vi "DIO_PanelSim_Global.vi"(0 "menu":T4=enum."set value", 5 "DIO Channel":T3=enum."DIO 1", 7 "pulse Length":dbl format="%#.4f", 9 "Value Set":bool, 11 "error in (no error)":errorcluster, 12 "String Value":string) -> (10 "DIO new":T1={"type"="DIO", "device"="", "name"="", "data"={"<init"=FALSE, "<>value"=FALSE, "<pulse_length"=0, "<input"=FALSE}}, 15 "error out":errorcluster)   [LabVIEW 2019]
doc: "This is used to set and get the last motor output values. This is needed for simulation, since we cannot read these values from the hardware.\n\nThis software is licensed. Open the labview\\readme\\WPI Robotics Library Open Source License.txt file for more information."
uses:
  DIO data proto.ctl
  DIO proto.ctl
  <vilib>/Rock Robotics/SystemInterfaces/DIO/FPGA_DIOChannel.ctl
  DIO Update Ops.ctl
panel:
  out "All Values":T1[](array[typedef])
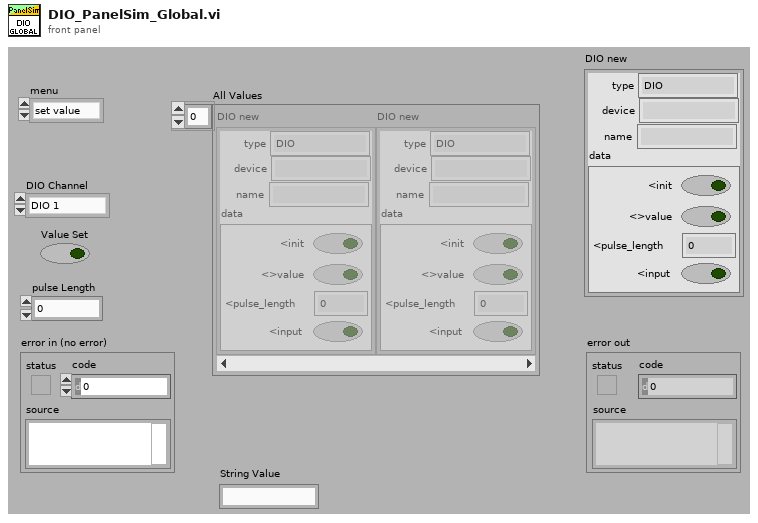
[diagram p1: front panel]
types:
  T1 = typedef "DIO proto.ctl" = cluster{"type":string, "device":string, "name":string, "data":T2}
  T2 = typedef "DIO data proto.ctl" = cluster{"<init":bool, "<>value":bool, "<pulse_length":i32, "<input":bool}
  T3 = typedef "FPGA_DIOChannel.ctl" = enum8{"DIO 0", "DIO 1", "DIO 2", "DIO 3", "DIO 4", "DIO 5", "DIO 6", "DIO 7", "DIO 8", "DIO 9", "DIO MXP 0", "DIO MXP 1", "DIO MXP 2", "DIO MXP 3", "DIO MXP 4", "DIO MXP 5", "DIO MXP 6", "DIO MXP 7", "DIO MXP 8", "DIO MXP 9", "DIO MXP 10", "DIO MXP 11", "DIO MXP 12", "DIO MXP 13", "DIO MXP 14", "DIO MXP 15", "SPI Port CS1", "SPI Port CS2", "SPI Port CS3", "SPI Port MISO", "SPI Port MOSI", "Invalid"}
  T4 = typedef "DIO Update Ops.ctl" = enum16{"set init", "set value", "set pulse_length", "set input", "get", "delete", "JSON update", "set name", "transmit initial", "reset"}
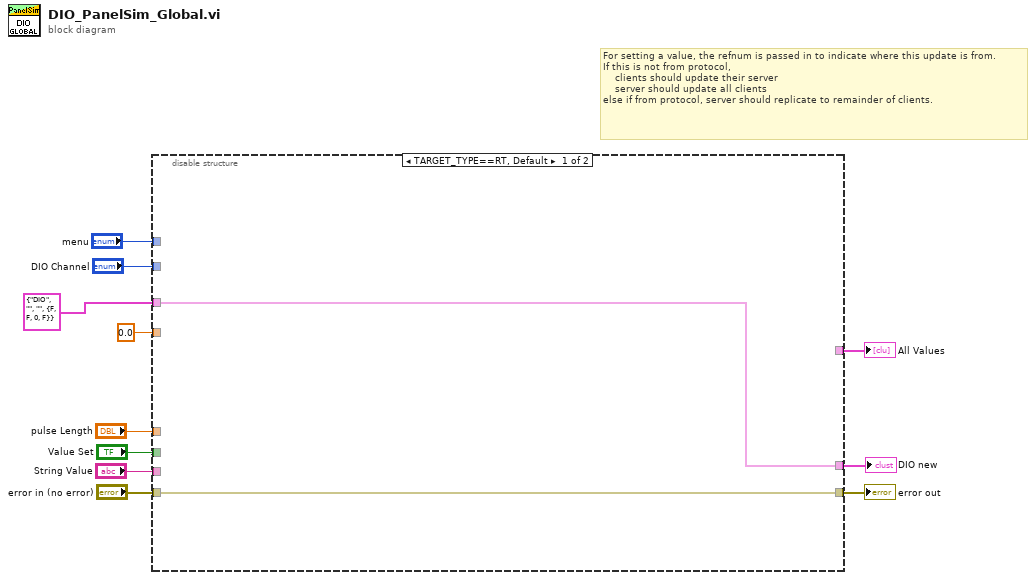
[diagram p0: block diagram]
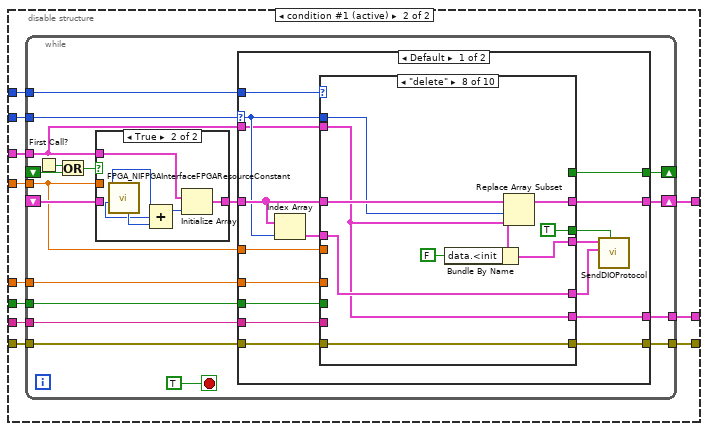
[diagram p2: hidden frame]
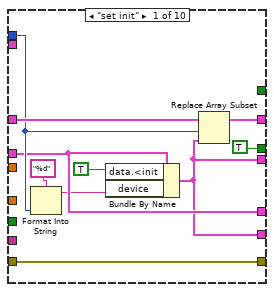
[diagram p3: hidden frame]
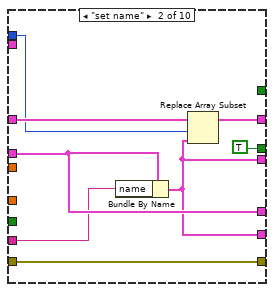
[diagram p4: hidden frame]
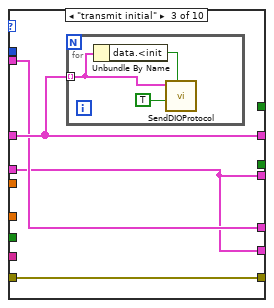
[diagram p5: hidden frame]
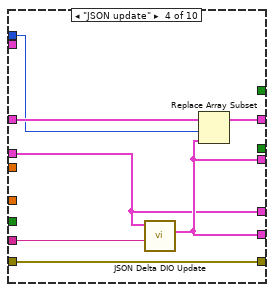
[diagram p6: hidden frame]
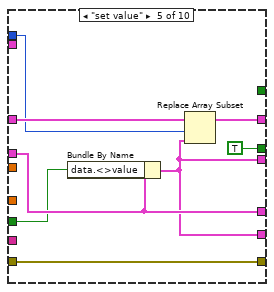
[diagram p7: hidden frame]
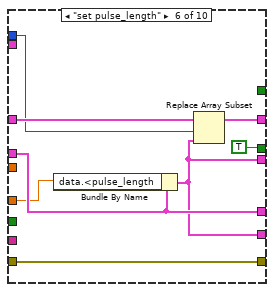
[diagram p8: hidden frame]
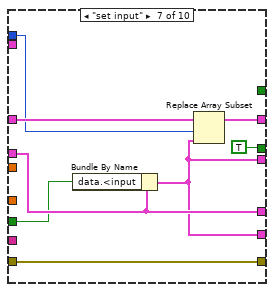
[diagram p9: hidden frame]
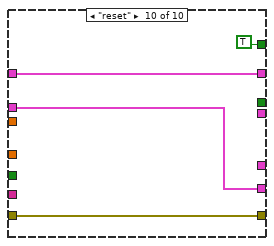
[diagram p11: hidden frame]
diagram:
  # "For setting a value, the refnum is passed in to indicate where this update is from.\nIf this is not from protocol,\n    clients should update their server\n    server should update all clients\nelse if from protocol, server should replicate to remainder of clients."
  n1 = disable-structure shown="TARGET_TYPE==RT, Default" {
    disable-tunnel: "menu" -> [_ w24]
    disable-tunnel: [w13 w23] -> w10
    disable-tunnel: "error in (no error)" -> [w13 w22]
    disable-tunnel: [_ w21] -> w8
    disable-tunnel: 0.0 ("Output") -> [_ w20]
    disable-tunnel: "Value Set" -> [_ w19]
    disable-tunnel: "DIO Channel" -> [_ w18]
    disable-tunnel: [w12 w17] -> w4
    disable-tunnel: T1 {"type"="DIO", "device"="", "name"="", "data"={"<init"=FALSE, "<>value"=FALSE, "<pulse_length"=0, "<input"=FALSE}} ("DIO new") -> [w12 w16]
    disable-tunnel: "String Value" -> [_ w15]
    disable-tunnel: "pulse Length" -> [_ w14]
    frame condition #0 {
    }
    frame condition #1 (active) {
      n2 = while {
        tunnel: w19 -> [w42]
        tunnel: w22 -> [w38]
        shift-right: [w41] -> w21
        shift-left: _ -> [w34]
        tunnel: [w40] -> w17
        tunnel: w24 -> [w39]
        tunnel: [w37] -> w23
        tunnel: w18 -> [w32]
        tunnel: w20 -> [w33]
        tunnel: w16 -> [w31]
        tunnel: w15 -> [w30]
        tunnel: w14 -> [w29]
        shift-right: [w25] -> _
        shift-left: _ -> [w26]
        stop <- TRUE stop-if-true
        n3 = First Call?() -> (First Call?: T/F=w27:bool)
        n4 = Or(x=w27, y=w26) -> (x .or. y?=w28:bool)
        n5 = case shown="True" w28 {
          tunnel: [w135 w141] -> w35
          tunnel: w34 -> [w135 _]
          tunnel: w33 -> [_ _]
          tunnel: w31 -> [_ w140]
          frame False {
          }
          frame True {
            n6 = call <vilib>:"FPGA_NIFPGAInterfaceFPGAResourceConstant.vi"() -> ("NumberOfDIOOnboard"=w138:u32, "NumberOfSPIDigitalPins"=w136:i32, "NumberOfSharedMXPpins"=w137:u32)  [unwired: 9 out]
            n7 = Compound Arithmetic op=ADD(w137, w136, w138) -> (w139:u32)
            n8 = Initialize Array(w140, w139) -> (w141:T1[])
          }
        }
        n9 = case shown="Default" w32 {
          selector: w32 -> [w51 _]
          tunnel: w42 -> [w59 _]
          tunnel: [w58 w134] -> w41
          tunnel: [w57 w132] -> w40
          tunnel: w39 -> [w56 _]
          tunnel: w38 -> [w55 w133]
          tunnel: [w54 w133] -> w37
          tunnel: w35 -> [w53 w134]
          tunnel: w33 -> [w52 _]
          tunnel: w31 -> [w49 w132]
          tunnel: w30 -> [w48 _]
          tunnel: w29 -> [w44 _]
          tunnel: [w43 _] -> w25
          frame Default {
            n10 = Index Array(array=w53, index=w51) -> (element=w50:T1)
            n11 = case shown="\"delete\"" w56 {
              tunnel: w59 -> [_ _ _ _ w93 _ w108 _ _ _]
              tunnel: [w69 w77 w80 w91 w99 w107 w115 w123 w127 w131] -> w58
              tunnel: w53 -> [w67 w75 w80 w89 w97 w105 w113 w124 w127 w131]
              tunnel: [w60 w71 w78 w87 w92 w101 w109 w117 w125 w129] -> w57
              tunnel: [w68 w76 w81 w90 w98 w106 w114 w122 w126 w130] -> w54
              tunnel: w55 -> [w68 w76 w81 w90 w98 w106 w114 w122 w126 w130]
              tunnel: w51 -> [w64 w73 _ w88 w95 w103 w111 w119 _ _]
              tunnel: w52 -> [_ _ _ _ _ _ _ _ _ _]
              tunnel: [w60 w71 w78 w87 w92 w101 w109 w118 _ _] -> w45
              tunnel: [w63 w72 w79 w85 w94 w102 w110 w120 _ _] -> w46
              tunnel: [TRUE TRUE _ _ TRUE TRUE TRUE TRUE _ _] -> w47
              tunnel: w50 -> [w63 w72 w78 w85 w94 w102 w110 w120 w125 w129]
              tunnel: w49 -> [_ _ w79 _ _ _ _ w117 _ _]
              tunnel: w48 -> [_ w70 _ w86 _ _ _ _ _ _]
              tunnel: w44 -> [_ _ _ _ _ w100 _ _ _ _]
              tunnel: [_ _ _ _ _ _ _ _ _ TRUE] -> w43
              frame "set init" {
                n12 = Format Into String(format string="%d", w64) -> (resulting string=w61:string)  [unwired: 2 in, 1 out]
                n13 = Bundle By Name(cluster=w63, "data.<init"=TRUE, "device"=w61) -> (w60:T1)
                n14 = Replace Array Subset(array=w67, new element=w60, index=w64) -> (w69:T1[])
              }
              frame "set name" {
                n15 = Bundle By Name(cluster=w72, "name"=w70) -> (w71:T1)
                n16 = Replace Array Subset(array=w75, new element=w71, index=w73) -> (w77:T1[])
              }
              frame "transmit initial" {
                n17 = for {
                  tunnel: w80 -> [w83] mode=indexing
                  n18 = Unbundle By Name(w83) -> ("data.<init"=w84:bool)
                  n19 = call "SendDIOProtocol.vi"("Send"=w84, "Initiualize"=TRUE, "DIO new"=w83) -> ()  [unwired: 9 in]
                }
              }
              frame "JSON update" {
                n20 = call "JSON Delta DIO Update.vi"("Delta JSON"=w86, "input"=w85) -> ("ouotput"=w87:T1)  [unwired: 8 in, 1 out]
                n21 = Replace Array Subset(array=w89, new element=w87, index=w88) -> (w91:T1[])
              }
              frame "set value" {
                n22 = Bundle By Name(cluster=w94, "data.<>value"=w93) -> (w92:T1)
                n23 = Replace Array Subset(array=w97, new element=w92, index=w95) -> (w99:T1[])
              }
              frame "set pulse_length" {
                n24 = Bundle By Name(cluster=w102, "data.<pulse_length"=w100) -> (w101:T1)
                n25 = Replace Array Subset(array=w105, new element=w101, index=w103) -> (w107:T1[])
              }
              frame "set input" {
                n26 = Bundle By Name(cluster=w110, "data.<input"=w108) -> (w109:T1)
                n27 = Replace Array Subset(array=w113, new element=w109, index=w111) -> (w115:T1[])
              }
              frame "delete" {
                n28 = Bundle By Name(cluster=w117, "data.<init"=FALSE) -> (w118:T1)
                n29 = Replace Array Subset(array=w124, new element=w117, index=w119) -> (w123:T1[])
              }
              frame "get" {
              }
              frame "reset" {
              }
            }
            n30 = call "SendDIOProtocol.vi"("Send"=w47, "DIO old"=w46, "DIO new"=w45) -> ()  [unwired: 9 in]
          }
          frame "Invalid" {
            # "Do nothing if \nchannel is Invalid."
          }
        }
      }
    }
  }
  "error out" <- w10
  "All Values" <- w8
  "DIO new" <- w4
